vi "Main.vi"(7 "sweep rate, /min":dbl=0.2, 8 "sweep to:":dbl=-0.5, 9 "sweep":T3(radio)=enum."time_sweep") -> ()   [LabVIEW 2017] (continued)
                    n3022 = property on="2336A_addr_step" class="VISAName"() -> ("Value"=w3898:refnum<visa-resource-name>)  [unwired: 2 in, 2 out]
                    n3023 = Subtract(x=w3897, y=w3899) -> (x-y=w3900:dbl)
                    n3024 = Divide(x=w3900, y=w3896) -> (x/y=w3901:dbl)
                    n3025 = for {
                      N: w3896 -> [_]
                      tunnel: w3899 -> [w3911]
                      tunnel: w3901 -> [w3910]
                      tunnel: w3898 -> [w3907]
                      i -> [w3906]
                      n3026 = Increment(x=w3906) -> (x+1=w3905:i32)
                      n3027 = Multiply(x=w3910, y=w3905) -> (x*y=w3909:dbl)
                      n3028 = Add(x=w3909, y=w3911) -> (x+y=w3902:dbl)
                      n3029 = call "setLevel.vi"("VISA resource name 2"=w3907, "Source"=Source."Voltage", "Channel"=Channel."a", "SourceLevel"=w3902) -> ("VISA resource name"=w3903:refnum<visa-resource-name>)  [unwired: 1 in, 2 out]
                      n3030 = Wait (ms)(milliseconds to wait=u32 12) -> ()  [unwired: 1 out]
                      n3031 = property on="Current Step Value" class="DigNum (strict)"("Value"=w3902) -> ()  [unwired: 2 in, 2 out]
                      n3032 = case shown="True" "diagonal step" {
                        tunnel: w3902 -> [_ w3921]
                        tunnel: w3903 -> [_ w3914]
                        frame False {
                        }
                        frame True {
                          n3033 = Multiply(x=w3921, y="Step Slope") -> (x*y=w3919:dbl)
                          n3034 = Add(x=w3919, y="Step Offset") -> (x+y=w3915:dbl)
                          n3035 = call "setLevel.vi"("VISA resource name 2"=w3914, "Source"=Source."Voltage", "Channel"=Channel."b", "SourceLevel"=w3915) -> ()  [unwired: 1 in, 3 out]
                        }
                      }
                    }
                  }
                  frame "Radio Selection 5" {
                    # "sweep voltage on 2636a smua"
                    n3036 = property on="Step Channel" class="DigNum (strict)"() -> ("Value"=w3925:dbl)  [unwired: 2 in, 2 out]
                    n3037 = property on="Mini steps" class="DigNum (strict)"() -> ("Value"=w3922:dbl)  [unwired: 2 in, 2 out]
                    n3038 = property on="2336A_addr_step" class="VISAName"() -> ("Value"=w3924:refnum<visa-resource-name>)  [unwired: 2 in, 2 out]
                    n3039 = Subtract(x=w3923, y=w3925) -> (x-y=w3926:dbl)
                    n3040 = Divide(x=w3926, y=w3922) -> (x/y=w3927:dbl)
                    n3041 = for {
                      N: w3922 -> [_]
                      tunnel: w3925 -> [w3937]
                      tunnel: w3927 -> [w3936]
                      tunnel: w3924 -> [w3933]
                      i -> [w3932]
                      n3042 = Increment(x=w3932) -> (x+1=w3931:i32)
                      n3043 = Multiply(x=w3936, y=w3931) -> (x*y=w3935:dbl)
                      n3044 = Add(x=w3935, y=w3937) -> (x+y=w3929:dbl)
                      n3045 = call "setLevel.vi"("VISA resource name 2"=w3933, "Source"=Source."Voltage", "Channel"=Channel."b", "SourceLevel"=w3929) -> ("VISA resource name"=w3930:refnum<visa-resource-name>)  [unwired: 1 in, 2 out]
                      n3046 = Wait (ms)(milliseconds to wait=u32 12) -> ()  [unwired: 1 out]
                      n3047 = property on="diagonal step" class="Bool (strict)"() -> ("Value"=w3928:bool)  [unwired: 2 in, 2 out]
                      n3048 = property on="Current Step Value" class="DigNum (strict)"("Value"=w3929) -> ()  [unwired: 2 in, 2 out]
                      n3049 = case shown="True" w3928 {
                        tunnel: w3929 -> [_ w3947]
                        tunnel: w3930 -> [_ w3942]
                        frame False {
                        }
                        frame True {
                          n3050 = property on="Step Slope" class="DigNum (strict)"() -> ("Value"=w3941:dbl)  [unwired: 2 in, 2 out]
                          n3051 = property on="Step Offset" class="DigNum (strict)"() -> ("Value"=w3940:dbl)  [unwired: 2 in, 2 out]
                          n3052 = Multiply(x=w3947, y=w3941) -> (x*y=w3946:dbl)
                          n3053 = Add(x=w3946, y=w3940) -> (x+y=w3943:dbl)
                          n3054 = call "setLevel.vi"("VISA resource name 2"=w3942, "Source"=Source."Voltage", "Channel"=Channel."a", "SourceLevel"=w3943) -> ()  [unwired: 1 in, 3 out]
                        }
                      }
                    }
                  }
                  frame "Radio Selection 6", Default {
                    # "do not sweep, just time"
                  }
                  frame "Radio Selection 7" {
                    # "step magnetic field"
                    n3055 = stacked-sequence {
                      tunnel: w3948 -> [w3954 w3961 _]
                      frame #0 {
                        # "go to setpoint"
                        n3056 = Number To Decimal String(number="IPS120-10 addr_Step") -> (decimal integer string=w3949:string)  [unwired: 1 in]
                        n3057 = Number To Fractional String(number=w3954, width (-)=6, precision (6)=3) -> (F-format string=w3958:string)  [unwired: 1 in]
                        n3058 = Concatenate Strings("$J ", w3958) -> (w3957:string)
                        n3059 = GPIB Write(0:w3949, 1:w3957, 2:1) -> (6:w3950:errorcluster)  [unwired: 2 in, 1 out]
                        n3060 = GPIB Write(0:w3949, 1:"$A1", 2:1, 3:w3950) -> ()  [unwired: 1 in, 2 out]
                      }
                      frame #1 {
                        n3061 = while {
                          tunnel: w3961 -> [w3966]
                          stop <- w3962 stop-if-true
                          w3974 = 1
                          n3062 = local read "IPS120-10 addr_Step"() -> (w3969:u8)
                          n3063 = Number To Decimal String(number=w3969) -> (decimal integer string=w3975:string)  [unwired: 1 in]
                          n3064 = GPIB Write(0:w3975, 1:"R 7", 2:w3974) -> (6:w3970:errorcluster)  [unwired: 2 in, 1 out]
                          n3065 = GPIB Read(0:w3975, 1:200, 2:w3974, 3:w3970) -> (5:w3973:string)  [unwired: 1 in, 2 out]
                          n3066 = Fract/Exp String To Number(string=w3973, offset=w3974) -> (number=w3967:dbl)  [unwired: 2 in, 1 out]
                          n3067 = Wait (ms)(milliseconds to wait=u32 500) -> ()  [unwired: 1 out]
                          n3068 = Subtract(x=w3967, y=w3966) -> (x-y=w3965:dbl)
                          n3069 = Absolute Value(x=w3965) -> (abs(x)=w3964:dbl)
                          n3070 = Less Or Equal?(x=w3964, y=0.01) -> (x <= y?=w3962:bool)
                          "at field" <- w3962
                        }
                      }
                      frame #2 {
                        n3071 = Wait (ms)(milliseconds to wait=u32 5000) -> ()  [unwired: 1 out]
                      }
                    }
                  }
                  frame "Radio Selection 8" {
                    # "step temperature"
                    n3072 = stacked-sequence {
                      tunnel: w3977 -> [w3980 w3987]
                      frame #0 {
                        n3073 = Number To Decimal String(number="ITC503S addr_step") -> (decimal integer string=w3979:string)  [unwired: 1 in]
                        n3074 = Number To Fractional String(number=w3980, width (-)=5, precision (6)=4) -> (F-format string=w3984:string)  [unwired: 1 in]
                        n3075 = Concatenate Strings("$T ", w3984) -> (w3983:string)
                        n3076 = GPIB Write(0:w3979, 1:w3983, 2:3) -> ()  [unwired: 2 in, 2 out]
                      }
                      frame #1 {
                        n3077 = while {
                          tunnel: w3987 -> [w4003]
                          stop <- w3988 stop-if-true
                          w3994 = 1
                          n3078 = property on="ITC503S addr_step" class="DigNum (strict)"() -> ("Value"=w3990:u8)  [unwired: 2 in, 2 out]
                          n3079 = Number To Decimal String(number=w3990) -> (decimal integer string=w3997:string)  [unwired: 1 in]
                          n3080 = GPIB Write(0:w3997, 1:"$C3", 2:1) -> (6:w3998:errorcluster)  [unwired: 2 in, 1 out]
                          n3081 = GPIB Write(0:w3997, 1:"R3", 2:w3994, 3:w3998) -> (6:w4000:errorcluster)  [unwired: 1 in, 1 out]
                          n3082 = GPIB Read(0:w3997, 1:200, 2:w3994, 3:w4000) -> (5:w3999:string)  [unwired: 1 in, 2 out]
                          n3083 = Wait (ms)(milliseconds to wait=u32 500) -> ()  [unwired: 1 out]
                          n3084 = Fract/Exp String To Number(string=w3999, offset=w3994) -> (number=w3991:dbl)  [unwired: 2 in, 1 out]
                          n3085 = property on="Tolerance_Step" class="DigNum (strict)"() -> ("Value"=w3989:dbl)  [unwired: 2 in, 2 out]
                          n3086 = Subtract(x=w3991, y=w4003) -> (x-y=w4002:dbl)
                          n3087 = Absolute Value(x=w4002) -> (abs(x)=w4001:dbl)
                          n3088 = Less Or Equal?(x=w4001, y=w3989) -> (x <= y?=w3988:bool)
                          n3089 = property on="at field" class="Bool (strict)"("Value"=w3988) -> ()  [unwired: 2 in, 2 out]
                        }
                      }
                    }
                  }
                }
              }
              frame #1 {
                n3090 = property on="Current Step Value" class="DigNum (strict)"() -> ("Value"=w4008:dbl)  [unwired: 2 in, 2 out]
                n3091 = property on="Step Channel" class="DigNum (strict)"("Value"=w4008) -> ()  [unwired: 2 in, 2 out]
                n3092 = property on="Wait Between Step(s)" class="DigNum (strict)"() -> ("Value"=w4007:i32)  [unwired: 2 in, 2 out]
                n3093 = Multiply(x=w4007, y=1000) -> (x*y=w4005:i32)
                n3094 = Wait (ms)(milliseconds to wait=w4005) -> ()  [unwired: 1 out]
              }
              frame #2 {
                n3095 = Enqueue Element(queue=w4010, element="Start Sweep") -> ()  [unwired: 2 in, 3 out]
              }
            }
          }
          frame True {
            # "When step values are all finished"
            n3096 = Enqueue Element(queue=w4016, element="Idle") -> ()  [unwired: 2 in, 3 out]
            n3097 = property on="Start Mapping" class="Bool"("DisabledEnum"=T5."Enabled" ("Disabled")) -> ()  [unwired: 2 in, 2 out]
            n3098 = property on="Stop Mapping" class="Bool"("DisabledEnum"=T5."Disabled and Grayed Out" ("Disabled")) -> ()  [unwired: 2 in, 2 out]
            n3099 = property on="Sweep Direction" class="Str"("Value"="Finished!" ("Sweep Direction"), "Text.TextColor"=u32 16711680 ("Text.Text Colors:Text Color")) -> ()  [unwired: 2 in, 2 out]
          }
        }
      }
      frame "Quit" {
      }
    }
  }
  n3100 = while {
    tunnel: w3 -> [w4021]
    tunnel: w2 -> [w4019]
    tunnel: w1 -> [w4018]
    stop <- w4020 stop-if-true
    # "This loop is the producer loop."
    n3101 = event shown="[2] \"Linetrace or Mapping?\": Value Change" {
      selector: _ -> [_ _ _ _ _ _ _ _ _ _ _ _ _ _]
      dyn-events: _ -> [_ _ _ _ _ _ _ _ _ _ _ _ _ _]
      timeout: _ -> [_ _ _ _ _ _ _ _ _ _ _ _ _ _]
      tunnel: w4021 -> [_ w4023 _ w4033 _ _ w4136 w4139 w4146 w4154 w4159 w4163 _ _]
      tunnel: [_ _ _ "Quit" _ _ _ _ _ _ _ _ _ _] -> w4020
      tunnel: w4019 -> [_ _ _ _ _ _ _ _ _ _ _ _ _ _]
      tunnel: w4018 -> [_ _ _ _ _ _ _ _ _ _ _ _ _ w4203]
      event Timeout {
        n3102 = event-data() -> ()  [unwired: 1 in, 3 out]
      }
      event "Initialize": Value Change {
        n3103 = event-data() -> ()  [unwired: 1 in, 6 out]
        n3104 = Enqueue Element(queue=w4023, element="Idle") -> ()  [unwired: 2 in, 3 out]
      }
      event "Linetrace or Mapping?": Value Change {
        n3105 = event-data() -> ()  [unwired: 1 in, 1 out]
        n3106 = case shown="False" "Linetrace or Mapping?" {
          frame True {
            w4025 = T5."Enabled" ("Disabled")
            w4026 = T5."Disabled and Grayed Out" ("Disabled")
            n3107 = property on="Ramp\n Down" class="Bool"("DisabledEnum"=w4026) -> ()  [unwired: 2 in, 2 out]
            n3108 = property on="sweep" class="RadioBtnsControl (strict)"("DisabledEnum"=w4026) -> ()  [unwired: 2 in, 2 out]
            n3109 = property on="2182A 1 addr" class="DigNum (strict)"("DisabledEnum"=w4026) -> ()  [unwired: 2 in, 2 out]
            n3110 = property on="2182A 2 addr" class="DigNum (strict)"("DisabledEnum"=w4026) -> ()  [unwired: 2 in, 2 out]
            n3111 = property on="2182A 3 addr" class="DigNum (strict)"("DisabledEnum"=w4026) -> ()  [unwired: 2 in, 2 out]
            n3112 = property on="2182A 4 addr" class="DigNum (strict)"("DisabledEnum"=w4026) -> ()  [unwired: 2 in, 2 out]
            n3113 = property on="2400 1 addr" class="DigNum (strict)"("DisabledEnum"=w4026) -> ()  [unwired: 2 in, 2 out]
            n3114 = property on="IPS120-0 addr_sweep" class="DigNum (strict)"("DisabledEnum"=w4026) -> ()  [unwired: 2 in, 2 out]
            n3115 = property on="iTC_503_addr_sweep" class="DigNum (strict)"("DisabledEnum"=w4026) -> ()  [unwired: 2 in, 2 out]
            n3116 = property on="Sweep Down" class="Bool"("DisabledEnum"=w4026) -> ()  [unwired: 2 in, 2 out]
            n3117 = property on="SR830 2 addr" class="DigNum (strict)"("DisabledEnum"=w4026) -> ()  [unwired: 2 in, 2 out]
            n3118 = property on="SR830 3 addr" class="DigNum (strict)"("DisabledEnum"=w4026) -> ()  [unwired: 2 in, 2 out]
            n3119 = property on="2400 2 addr" class="DigNum (strict)"("DisabledEnum"=w4026) -> ()  [unwired: 2 in, 2 out]
            n3120 = property on="2400 3 addr" class="DigNum (strict)"("DisabledEnum"=w4026) -> ()  [unwired: 2 in, 2 out]
            n3121 = property on="2336A addr" class="VISAName"("DisabledEnum"=w4026) -> ()  [unwired: 2 in, 2 out]
            n3122 = property on="SR830 1 addr" class="DigNum (strict)"("DisabledEnum"=w4026) -> ()  [unwired: 2 in, 2 out]
            n3123 = property on="SR830 4 addr" class="DigNum (strict)"("DisabledEnum"=w4026) -> ()  [unwired: 2 in, 2 out]
            n3124 = property on="Ramp \nUp" class="Bool"("DisabledEnum"=w4026) -> ()  [unwired: 2 in, 2 out]
            n3125 = property on="Sweep Up" class="Bool"("DisabledEnum"=w4026) -> ()  [unwired: 2 in, 2 out]
            n3126 = property on="Tolerance_Sweep" class="DigNum (strict)"("DisabledEnum"=w4026) -> ()  [unwired: 2 in, 2 out]
            n3127 = property on="Continuous Sweep" class="Bool (strict)"("DisabledEnum"=w4026) -> ()  [unwired: 2 in, 2 out]
            n3128 = property on="Continuous Sweep" class="Bool (strict)"("Value"=FALSE ("Continuous Sweep")) -> ()  [unwired: 2 in, 2 out]
            n3129 = property on="MappingName" class="Str"("Visible"=TRUE) -> ()  [unwired: 2 in, 2 out]
            n3130 = property on="step" class="RadioBtnsControl (strict)"("DisabledEnum"=w4025) -> ()  [unwired: 2 in, 2 out]
            n3131 = property on="diagonal step" class="Bool (strict)"("DisabledEnum"=w4025) -> ()  [unwired: 2 in, 2 out]
            n3132 = property on="Step Offset" class="DigNum (strict)"("DisabledEnum"=w4025) -> ()  [unwired: 2 in, 2 out]
            n3133 = property on="Step Slope" class="DigNum (strict)"("DisabledEnum"=w4025) -> ()  [unwired: 2 in, 2 out]
            n3134 = property on="FieldRate(T/min)" class="DigNum (strict)"("DisabledEnum"=w4025) -> ()  [unwired: 2 in, 2 out]
            n3135 = property on="wait between sweeps(s)" class="DigNum (strict)"("DisabledEnum"=w4025) -> ()  [unwired: 2 in, 2 out]
            n3136 = property on="2336A_addr_step" class="VISAName"("DisabledEnum"=w4025) -> ()  [unwired: 2 in, 2 out]
            n3137 = property on="Start Mapping" class="Bool"("DisabledEnum"=w4025) -> ()  [unwired: 2 in, 2 out]
            n3138 = property on="2400_1_addr_step" class="DigNum (strict)"("DisabledEnum"=w4025) -> ()  [unwired: 2 in, 2 out]
            n3139 = property on="Tolerance_Step" class="DigNum (strict)"("DisabledEnum"=w4025) -> ()  [unwired: 2 in, 2 out]
            n3140 = property on="Wait Between Step(s)" class="DigNum (strict)"("DisabledEnum"=w4025) -> ()  [unwired: 2 in, 2 out]
            n3141 = property on="2400_2_addr_step" class="DigNum (strict)"("DisabledEnum"=w4025) -> ()  [unwired: 2 in, 2 out]
            n3142 = property on="IPS120-10 addr_Step" class="DigNum (strict)"("DisabledEnum"=w4025) -> ()  [unwired: 2 in, 2 out]
            n3143 = property on="ITC503S addr_step" class="DigNum (strict)"("DisabledEnum"=w4025) -> ()  [unwired: 2 in, 2 out]
          }
          frame False {
            w4029 = T5."Disabled and Grayed Out" ("Disabled")
            w4030 = T5."Enabled" ("Disabled")
            n3144 = property on="Ramp\n Down" class="Bool"("DisabledEnum"=w4030) -> ()  [unwired: 2 in, 2 out]
            n3145 = property on="sweep" class="RadioBtnsControl (strict)"("DisabledEnum"=w4030) -> ()  [unwired: 2 in, 2 out]
            n3146 = property on="2182A 1 addr" class="DigNum (strict)"("DisabledEnum"=w4030) -> ()  [unwired: 2 in, 2 out]
            n3147 = property on="2182A 2 addr" class="DigNum (strict)"("DisabledEnum"=w4030) -> ()  [unwired: 2 in, 2 out]
            n3148 = property on="2182A 3 addr" class="DigNum (strict)"("DisabledEnum"=w4030) -> ()  [unwired: 2 in, 2 out]
            n3149 = property on="2182A 4 addr" class="DigNum (strict)"("DisabledEnum"=w4030) -> ()  [unwired: 2 in, 2 out]
            n3150 = property on="2400 1 addr" class="DigNum (strict)"("DisabledEnum"=w4030) -> ()  [unwired: 2 in, 2 out]
            n3151 = property on="IPS120-0 addr_sweep" class="DigNum (strict)"("DisabledEnum"=w4030) -> ()  [unwired: 2 in, 2 out]
            n3152 = property on="iTC_503_addr_sweep" class="DigNum (strict)"("DisabledEnum"=w4030) -> ()  [unwired: 2 in, 2 out]
            n3153 = property on="Sweep Down" class="Bool"("DisabledEnum"=w4030) -> ()  [unwired: 2 in, 2 out]
            n3154 = property on="SR830 2 addr" class="DigNum (strict)"("DisabledEnum"=w4030) -> ()  [unwired: 2 in, 2 out]
            n3155 = property on="SR830 3 addr" class="DigNum (strict)"("DisabledEnum"=w4030) -> ()  [unwired: 2 in, 2 out]
            n3156 = property on="2400 2 addr" class="DigNum (strict)"("DisabledEnum"=w4030) -> ()  [unwired: 2 in, 2 out]
            n3157 = property on="2400 3 addr" class="DigNum (strict)"("DisabledEnum"=w4030) -> ()  [unwired: 2 in, 2 out]
            n3158 = property on="2336A addr" class="VISAName"("DisabledEnum"=w4030) -> ()  [unwired: 2 in, 2 out]
            n3159 = property on="SR830 1 addr" class="DigNum (strict)"("DisabledEnum"=w4030) -> ()  [unwired: 2 in, 2 out]
            n3160 = property on="SR830 4 addr" class="DigNum (strict)"("DisabledEnum"=w4030) -> ()  [unwired: 2 in, 2 out]
            n3161 = property on="Ramp \nUp" class="Bool"("DisabledEnum"=w4030) -> ()  [unwired: 2 in, 2 out]
            n3162 = property on="Sweep Up" class="Bool"("DisabledEnum"=w4030) -> ()  [unwired: 2 in, 2 out]
            n3163 = property on="Tolerance_Sweep" class="DigNum (strict)"("DisabledEnum"=w4030) -> ()  [unwired: 2 in, 2 out]
            n3164 = property on="Continuous Sweep" class="Bool (strict)"("DisabledEnum"=w4030) -> ()  [unwired: 2 in, 2 out]
            n3165 = property on="MappingName" class="Str"("Visible"=FALSE) -> ()  [unwired: 2 in, 2 out]
            n3166 = property on="step" class="RadioBtnsControl (strict)"("DisabledEnum"=w4029) -> ()  [unwired: 2 in, 2 out]
            n3167 = property on="diagonal step" class="Bool (strict)"("DisabledEnum"=w4029) -> ()  [unwired: 2 in, 2 out]
            n3168 = property on="Step Offset" class="DigNum (strict)"("DisabledEnum"=w4029) -> ()  [unwired: 2 in, 2 out]
            n3169 = property on="Step Slope" class="DigNum (strict)"("DisabledEnum"=w4029) -> ()  [unwired: 2 in, 2 out]
            n3170 = property on="wait between sweeps(s)" class="DigNum (strict)"("DisabledEnum"=w4029) -> ()  [unwired: 2 in, 2 out]
            n3171 = property on="2336A_addr_step" class="VISAName"("DisabledEnum"=w4029) -> ()  [unwired: 2 in, 2 out]
            n3172 = property on="Start Mapping" class="Bool"("DisabledEnum"=w4029) -> ()  [unwired: 2 in, 2 out]
            n3173 = property on="2400_1_addr_step" class="DigNum (strict)"("DisabledEnum"=w4029) -> ()  [unwired: 2 in, 2 out]
            n3174 = property on="Wait Between Step(s)" class="DigNum (strict)"("DisabledEnum"=w4029) -> ()  [unwired: 2 in, 2 out]
            n3175 = property on="2400_2_addr_step" class="DigNum (strict)"("DisabledEnum"=w4029) -> ()  [unwired: 2 in, 2 out]
            n3176 = property on="FieldRate(T/min)" class="DigNum (strict)"("DisabledEnum"=w4029) -> ()  [unwired: 2 in, 2 out]
            n3177 = property on="IPS120-10 addr_Step" class="DigNum (strict)"("DisabledEnum"=w4029) -> ()  [unwired: 2 in, 2 out]
            n3178 = property on="ITC503S addr_step" class="DigNum (strict)"("DisabledEnum"=w4029) -> ()  [unwired: 2 in, 2 out]
            n3179 = property on="Tolerance_Step" class="DigNum (strict)"("DisabledEnum"=w4029) -> ()  [unwired: 2 in, 2 out]
          }
        }
      }
      event "Quit": Value Change {
        n3180 = event-data() -> ()  [unwired: 1 in, 6 out]
        n3181 = Flush Queue(queue=w4033) -> (queue out=w4032:refnum<queue>)  [unwired: 1 in, 2 out]
        n3182 = Enqueue Element(queue=w4032, element="Quit") -> ()  [unwired: 2 in, 3 out]
      }
      event "Populate step table?": Value Change {
        n3183 = event-data() -> ()  [unwired: 1 in, 6 out]
        n3184 = stacked-sequence {
          frame #0 {
            n3185 = property on="Step values" class="Tbl (strict)"("Active Cell"=cluster{"Row":i32, "Column":i32} {"Row"=-2, "Column"=-2}, "Cell BG Color"=u32 16448250 ("Active Cell:Cell Background Color")) -> ()  [unwired: 2 in, 2 out]
          }
          frame #1 {
            n3186 = Subtract(x="from", y="to") -> (x-y=w4047:dbl)
            n3187 = Divide(x=w4047, y="step") -> (x/y=w4046:dbl)
            n3188 = Sign(1:w4047) -> (0:w4050:dbl)
            n3189 = Absolute Value(x=w4046) -> (abs(x)=w4045:dbl)
            n3190 = Negate(x=w4050) -> (-x=w4042:dbl)
            n3191 = Round Toward -Infinity(1:w4045) -> (0:w4044:dbl)
            n3192 = Increment(x=w4044) -> (x+1=w4043:dbl)
            n3193 = for {
              N: w4043 -> [_]
              tunnel: "from" -> [w4056]
              tunnel: w4042 -> [w4057]
              tunnel: "step" -> [w4059]
              tunnel: [w4053] -> w4048 mode=indexing
              i -> [w4051]
              n3194 = Multiply(x=w4059, y=w4051) -> (x*y=w4058:dbl)
              n3195 = Multiply(x=w4057, y=w4058) -> (x*y=w4055:dbl)
              n3196 = Add(x=w4056, y=w4055) -> (x+y=w4054:dbl)
              n3197 = Number To Fractional String(number=w4054, precision (6)=i16 6) -> (F-format string=w4053:string)  [unwired: 2 in]
            }
            n3198 = Build Array(w4048) -> (w4049:string[][])
            n3199 = Transpose 2D Array(2D array=w4049) -> (transposed array=w4041:string[][])
            n3200 = property on="Step values" class="Tbl (strict)"("Value"=w4041) -> ()  [unwired: 2 in, 2 out]
          }
          frame #2 {
            n3201 = property on="upper limit" class="DigNum (strict)"() -> ("Value"=w4089:dbl)  [unwired: 2 in, 2 out]
            n3202 = property on="lower limit" class="DigNum (strict)"() -> ("Value"=w4090:dbl)  [unwired: 2 in, 2 out]
            n3203 = Subtract(x=w4090, y=w4089) -> (x-y=w4088:dbl)
            n3204 = property on="Down Rate" class="DigNum (strict)"() -> ("Value"=w4085:dbl)  [unwired: 2 in, 2 out]
            n3205 = property on="Up Rate" class="DigNum (strict)"() -> ("Value"=w4087:dbl)  [unwired: 2 in, 2 out]
            n3206 = Absolute Value(x=w4088) -> (abs(x)=w4086:dbl)
            n3207 = property on="step" class="RadioBtnsControl (strict)"() -> ("Value"=w4061:T2)  [unwired: 2 in, 2 out]
            n3208 = Divide(x=w4086, y=w4087) -> (x/y=w4084:dbl)
            n3209 = Divide(x=w4086, y=w4085) -> (x/y=w4083:dbl)
            n3210 = case shown="\"Radio Selection 7\"" w4061 {
              tunnel: [w4091 0.0] -> w4060
              frame "Radio Selection 7" {
                n3211 = property on="step" class="DigNum (strict)"() -> ("Value"=w4095:dbl)  [unwired: 2 in, 2 out]
                n3212 = property on="FieldRate(T/min)" class="DigNum (strict)"() -> ("Value"=w4094:dbl)  [unwired: 2 in, 2 out]
                n3213 = Divide(x=w4095, y=w4094) -> (x/y=w4093:dbl)
                n3214 = Multiply(x=w4093, y=60.0) -> (x*y=w4091:dbl)
              }
              frame "Radio Selection 1".."Radio Selection 8", Default {
              }
            }
            n3215 = property on="Wait Between Step(s)" class="DigNum (strict)"() -> ("Value"=w4080:i32)  [unwired: 2 in, 2 out]
            n3216 = Add(x=w4084, y=w4083) -> (x+y=w4082:dbl)
            n3217 = Multiply(x=w4082, y=60.0) -> (x*y=w4081:dbl)
            n3218 = property on="wait between sweeps(s)" class="DigNum (strict)"() -> ("Value"=w4078:u32)  [unwired: 2 in, 2 out]
            n3219 = Add(x=w4081, y=w4080) -> (x+y=w4079:dbl)
            n3220 = property on="Step values" class="Tbl (strict)"() -> ("Value"=w4074:string[][])  [unwired: 2 in, 2 out]
            n3221 = Array Size(array=w4074) -> (size(s)=w4073:i32[])
            n3222 = Add(x=w4079, y=w4078) -> (x+y=w4063:dbl)
            n3223 = Index Array(array=w4073, index=0) -> (element=w4072:i32)
            n3224 = Add(x=w4063, y=w4060) -> (x+y=w4062:dbl)
            n3225 = Get Date/Time In Seconds() -> (seconds since 1Jan1904=w4077:timestamp)
            n3226 = Multiply(x=w4072, y=w4062) -> (x*y=w4076:dbl)
            n3227 = Add(x=w4076, y=w4077) -> (x+y=w4071:timestamp)
            n3228 = Quotient & Remainder(x=w4076, y=3600.0) -> (x-y*floor(x/y)=w4075:dbl, floor(x/y)=w4070:dbl)
            n3229 = Quotient & Remainder(x=w4075, y=60.0) -> (x-y*floor(x/y)=w4068:dbl, floor(x/y)=w4069:dbl)
            n3230 = property on="SS" class="DigNum (strict)"("Value"=w4068) -> ()  [unwired: 2 in, 2 out]
            n3231 = property on="MM:" class="DigNum (strict)"("Value"=w4069) -> ()  [unwired: 2 in, 2 out]
            n3232 = property on="HH:" class="DigNum (strict)"("Value"=w4070) -> ()  [unwired: 2 in, 2 out]
            n3233 = property on="Finish Time" class="AbsTime (strict)"("Value"=w4071) -> ()  [unwired: 2 in, 2 out]
          }
        }
      }
      event "EstimateTime": Value Change {
        n3234 = event-data() -> ()  [unwired: 1 in, 6 out]
        n3235 = property on="upper limit" class="DigNum (strict)"() -> ("Value"=w4126:dbl)  [unwired: 2 in, 2 out]
        n3236 = property on="lower limit" class="DigNum (strict)"() -> ("Value"=w4127:dbl)  [unwired: 2 in, 2 out]
        n3237 = Subtract(x=w4127, y=w4126) -> (x-y=w4125:dbl)
        n3238 = property on="Down Rate" class="DigNum (strict)"() -> ("Value"=w4122:dbl)  [unwired: 2 in, 2 out]
        n3239 = property on="Up Rate" class="DigNum (strict)"() -> ("Value"=w4124:dbl)  [unwired: 2 in, 2 out]
        n3240 = Absolute Value(x=w4125) -> (abs(x)=w4123:dbl)
        n3241 = property on="step" class="RadioBtnsControl (strict)"() -> ("Value"=w4100:T2)  [unwired: 2 in, 2 out]
        n3242 = Divide(x=w4123, y=w4124) -> (x/y=w4121:dbl)
        n3243 = Divide(x=w4123, y=w4122) -> (x/y=w4120:dbl)
        n3244 = case shown="\"Radio Selection 7\"" w4100 {
          tunnel: [w4128 0.0] -> w4098
          frame "Radio Selection 7" {
            n3245 = property on="step" class="DigNum (strict)"() -> ("Value"=w4132:dbl)  [unwired: 2 in, 2 out]
            n3246 = property on="FieldRate(T/min)" class="DigNum (strict)"() -> ("Value"=w4131:dbl)  [unwired: 2 in, 2 out]
            n3247 = Divide(x=w4132, y=w4131) -> (x/y=w4130:dbl)
            n3248 = Multiply(x=w4130, y=60.0) -> (x*y=w4128:dbl)
          }
          frame "Radio Selection 1".."Radio Selection 8", Default {
          }
        }
        n3249 = property on="Wait Between Step(s)" class="DigNum (strict)"() -> ("Value"=w4117:i32)  [unwired: 2 in, 2 out]
        n3250 = Add(x=w4121, y=w4120) -> (x+y=w4119:dbl)
        n3251 = Multiply(x=w4119, y=60.0) -> (x*y=w4118:dbl)
        n3252 = property on="wait between sweeps(s)" class="DigNum (strict)"() -> ("Value"=w4115:u32)  [unwired: 2 in, 2 out]
        n3253 = Add(x=w4118, y=w4117) -> (x+y=w4116:dbl)
        n3254 = Add(x=w4116, y=w4115) -> (x+y=w4099:dbl)
        n3255 = property on="Step values" class="Tbl (strict)"() -> ("Value"=w4108:string[][])  [unwired: 2 in, 2 out]
        n3256 = Add(x=w4099, y=w4098) -> (x+y=w4097:dbl)
        n3257 = Array Size(array=w4108) -> (size(s)=w4107:i32[])
        n3258 = Index Array(array=w4107, index=0) -> (element=w4105:i32)
        n3259 = Get Date/Time In Seconds() -> (seconds since 1Jan1904=w4114:timestamp)
        n3260 = Multiply(x=w4105, y=w4097) -> (x*y=w4113:dbl)
        n3261 = Add(x=w4113, y=w4114) -> (x+y=w4104:timestamp)
        n3262 = Quotient & Remainder(x=w4113, y=3600.0) -> (x-y*floor(x/y)=w4112:dbl, floor(x/y)=w4103:dbl)
        n3263 = Quotient & Remainder(x=w4112, y=60.0) -> (x-y*floor(x/y)=w4101:dbl, floor(x/y)=w4102:dbl)
        n3264 = property on="SS" class="DigNum (strict)"("Value"=w4101) -> ()  [unwired: 2 in, 2 out]
        n3265 = property on="MM:" class="DigNum (strict)"("Value"=w4102) -> ()  [unwired: 2 in, 2 out]
        n3266 = property on="HH:" class="DigNum (strict)"("Value"=w4103) -> ()  [unwired: 2 in, 2 out]
        n3267 = property on="Finish Time" class="AbsTime (strict)"("Value"=w4104) -> ()  [unwired: 2 in, 2 out]
      }
      event "Stop Mapping": Value Change {
        n3268 = event-data() -> ()  [unwired: 1 in, 6 out]
        n3269 = Flush Queue(queue=w4136) -> (queue out=w4137:refnum<queue>)  [unwired: 1 in, 2 out]
        n3270 = Enqueue Element(queue=w4137, element="Idle") -> ()  [unwired: 2 in, 3 out]
        n3271 = property on="Start Mapping" class="Bool"("DisabledEnum"=T5."Enabled" ("Disabled")) -> ()  [unwired: 2 in, 2 out]
        n3272 = property on="Stop Mapping" class="Bool"("DisabledEnum"=T5."Disabled and Grayed Out" ("Disabled")) -> ()  [unwired: 2 in, 2 out]
      }
      event "Sweep Down": Value Change {
        n3273 = event-data() -> ()  [unwired: 1 in, 6 out]
        n3274 = stacked-sequence {
          tunnel: w4139 -> [_ w4144]
          frame #0 {
            n3275 = property on="Down Rate" class="DigNum (strict)"() -> ("Value"=w4140:dbl)  [unwired: 2 in, 2 out]
            n3276 = property on="lower limit" class="DigNum (strict)"() -> ("Value"=w4141:dbl)  [unwired: 2 in, 2 out]
            n3277 = property on="sweep rate, /min" class="DigNum (strict)"("Value"=w4140) -> ()  [unwired: 2 in, 2 out]
            n3278 = property on="sweep to:" class="DigNum (strict)"("Value"=w4141) -> ()  [unwired: 2 in, 2 out]
            n3279 = property on="Sweep Down" class="Bool"("DisabledEnum"=T5."Disabled and Grayed Out" ("Disabled")) -> ()  [unwired: 2 in, 2 out]
          }
          frame #1 {
            n3280 = Flush Queue(queue=w4144) -> (queue out=w4143:refnum<queue>)  [unwired: 1 in, 2 out]
            n3281 = Enqueue Element(queue=w4143, element="Start Sweep") -> ()  [unwired: 2 in, 3 out]
          }
        }
      }
      event "Sweep Up": Value Change {
        n3282 = event-data() -> ()  [unwired: 1 in, 6 out]
        n3283 = stacked-sequence {
          tunnel: w4146 -> [_ w4151]
          frame #0 {
            w4147 = T5."Disabled and Grayed Out" ("Disabled")
            n3284 = property on="Up Rate" class="DigNum (strict)"() -> ("Value"=w4148:dbl)  [unwired: 2 in, 2 out]
            n3285 = property on="upper limit" class="DigNum (strict)"() -> ("Value"=w4149:dbl)  [unwired: 2 in, 2 out]
            n3286 = property on="sweep rate, /min" class="DigNum (strict)"("Value"=w4148) -> ()  [unwired: 2 in, 2 out]
            n3287 = property on="sweep to:" class="DigNum (strict)"("Value"=w4149) -> ()  [unwired: 2 in, 2 out]
            n3288 = property on="Sweep Down" class="Bool"("DisabledEnum"=w4147) -> ()  [unwired: 2 in, 2 out]
            n3289 = property on="Sweep Up" class="Bool"("DisabledEnum"=w4147) -> ()  [unwired: 2 in, 2 out]
          }
          frame #1 {
            n3290 = Flush Queue(queue=w4151) -> (queue out=w4150:refnum<queue>)  [unwired: 1 in, 2 out]
            n3291 = Enqueue Element(queue=w4150, element="Start Sweep") -> ()  [unwired: 2 in, 3 out]
          }
        }
      }
      event "Ramp\n Down": Value Change {
        n3292 = event-data() -> ()  [unwired: 1 in, 6 out]
        n3293 = Flush Queue(queue=w4154) -> (queue out=w4153:refnum<queue>)  [unwired: 1 in, 2 out]
        n3294 = property on="lower limit" class="DigNum (strict)"() -> ("Value"=w4157:dbl)  [unwired: 2 in, 2 out]
        n3295 = property on="Down Rate" class="DigNum (strict)"() -> ("Value"=w4156:dbl)  [unwired: 2 in, 2 out]
        n3296 = Enqueue Element(queue=w4153, element="Ramp To Limit") -> ()  [unwired: 2 in, 3 out]
        n3297 = property on="sweep to:" class="DigNum (strict)"("Value"=w4157) -> ()  [unwired: 2 in, 2 out]
        n3298 = property on="sweep rate, /min" class="DigNum (strict)"("Value"=w4156) -> ()  [unwired: 2 in, 2 out]
      }
      event "Ramp \nUp": Value Change {
        n3299 = event-data() -> ()  [unwired: 1 in, 6 out]
        n3300 = Flush Queue(queue=w4159) -> (queue out=w4158:refnum<queue>)  [unwired: 1 in, 2 out]
        n3301 = property on="Up Rate" class="DigNum (strict)"() -> ("Value"=w4160:dbl)  [unwired: 2 in, 2 out]
        n3302 = property on="upper limit" class="DigNum (strict)"() -> ("Value"=w4161:dbl)  [unwired: 2 in, 2 out]
        n3303 = Enqueue Element(queue=w4158, element="Ramp To Limit") -> ()  [unwired: 2 in, 3 out]
        n3304 = property on="sweep rate, /min" class="DigNum (strict)"("Value"=w4160) -> ()  [unwired: 2 in, 2 out]
        n3305 = property on="sweep to:" class="DigNum (strict)"("Value"=w4161) -> ()  [unwired: 2 in, 2 out]
      }
      event "Start Mapping": Value Change {
        n3306 = event-data() -> ()  [unwired: 1 in, 6 out]
        n3307 = stacked-sequence {
          tunnel: w4163 -> [_ _ _ w4194]
          frame #0 {
            n3308 = property on="Step values" class="Tbl (strict)"("Active Cell"=cluster{"Row":i32, "Column":i32} {"Row"=-2, "Column"=-2}, "Cell BG Color"=u32 16448250 ("Active Cell:Cell Background Color")) -> ()  [unwired: 2 in, 2 out]
          }
          frame #1 {
            n3309 = property on="lower limit" class="DigNum (strict)" props=["Value"]() -> ()  [unwired: 2 in, 3 out]
            n3310 = property on="Stop Mapping" class="Bool"("DisabledEnum"=T5."Enabled" ("Disabled")) -> ()  [unwired: 2 in, 2 out]
            n3311 = property on="upper limit" class="DigNum (strict)"() -> ("Value"=w4166:dbl)  [unwired: 2 in, 2 out]
            n3312 = property on="Down Rate" class="DigNum (strict)"() -> ("Value"=w4169:dbl)  [unwired: 2 in, 2 out]
            n3313 = property on="sweep to:" class="DigNum (strict)"("Value"=w4166) -> ()  [unwired: 2 in, 2 out]
            n3314 = property on="sweep rate, /min" class="DigNum (strict)"("Value"=w4169) -> ()  [unwired: 2 in, 2 out]
            n3315 = property on="Sweep Direction" class="Str"("Value"="Ramp Down" ("String"), "Text.TextColor"=u32 0 ("Text.Text Colors:Text Color")) -> ()  [unwired: 2 in, 2 out]
            n3316 = property on="Start Mapping" class="Bool"("DisabledEnum"=T5."Disabled and Grayed Out" ("Disabled")) -> ()  [unwired: 2 in, 2 out]
            n3317 = property on="Table Index" class="DigNum (strict)"("Value"=0.0 ("Table Index")) -> ()  [unwired: 2 in, 2 out]
          }
          frame #2 {
            # "Reserve two name strings for new mapping data file:\none for up\none for down"
            n3318 = property on="Data Folder" class="Path"() -> ("Value"=w4174:path)  [unwired: 2 in, 2 out]
            n3319 = stacked-sequence {
              tunnel: w4174 -> [w4179 w4188]
              tunnel: "MappingName" -> [w4177 w4186]
              frame #0 {
                # "Up mapping"
                n3320 = Concatenate Strings(w4177, "_up") -> (w4175:string)
                n3321 = call "AutoNamerDatExtraArtem.vi"("SweepType"=w4175, "Custom User Path"=w4179) -> ("String"=w4182:string, "Path"=w4183:path)  [unwired: 2 in]
                n3322 = Path To String(path=w4183) -> (string=w4181:string)
                n3323 = Concatenate Strings(w4181, "\\", w4182) -> (→"UpNameString":string)
              }
              frame #1 {
                # "Down mapping"
                n3324 = Concatenate Strings(w4186, "_down") -> (w4184:string)
                n3325 = call "AutoNamerDatExtraArtem.vi"("SweepType"=w4184, "Custom User Path"=w4188) -> ("String"=w4191:string, "Path"=w4192:path)  [unwired: 2 in]
                n3326 = Path To String(path=w4192) -> (string=w4190:string)
                n3327 = Concatenate Strings(w4190, "\\", w4191) -> (→"DownNameString":string)
              }
            }
          }
          frame #3 {
            n3328 = Flush Queue(queue=w4194) -> (queue out=w4193:refnum<queue>)  [unwired: 1 in, 2 out]
            n3329 = Enqueue Element(queue=w4193, element="Ramp To Limit") -> ()  [unwired: 2 in, 3 out]
          }
        }
      }
      event "Monitor": Value Change {
        n3330 = event-data() -> ()  [unwired: 1 in, 6 out]
        n3331 = case shown="False" "Monitor" {
          frame True {
            w4197 = TRUE ("Visible")
            n3332 = property on="Figure_axis" class="Arr (strict)"("Visible"=w4197) -> ()  [unwired: 2 in, 2 out]
            n3333 = property on="data" class="Arr (strict)"("Visible"=w4197) -> ()  [unwired: 2 in, 2 out]
            n3334 = property on="formula_variables" class="Arr (strict)"("Visible"=w4197) -> ()  [unwired: 2 in, 2 out]
          }
          frame False {
            w4198 = FALSE ("Visible")
            n3335 = property on="Figure_axis" class="Arr (strict)"("Visible"=w4198) -> ()  [unwired: 2 in, 2 out]
            n3336 = property on="formula_variables" class="Arr (strict)"("Visible"=w4198) -> ()  [unwired: 2 in, 2 out]
            n3337 = property on="data" class="Arr (strict)"("Visible"=w4198) -> ()  [unwired: 2 in, 2 out]
          }
        }
      }
      event "Lockin_Setup", "Cytec_Switch": Value Change {
        n3338 = event-data() -> ("CtlRef"=w4205:refnum<vi>)  [unwired: 1 in, 5 out]
        n3339 = property class="Bool"(reference=w4205) -> ("Label.Text"=w4204:string)  [unwired: 1 in, 2 out]
        n3340 = case shown="\"Cytec_Switch\", Default" w4204 {
          tunnel: w4203 -> [w4210 w4212]
          tunnel: [w4209 w4211] -> w4202
          frame "Cytec_Switch", Default {
            n3341 = Unbundle(w4210) -> ("vi reference"=w4209:refnum<vi>)  [unwired: 1 out]
          }
          frame "Lockin_Setup" {
            n3342 = Unbundle(w4212) -> ("vi reference"=w4211:refnum<vi>)  [unwired: 1 out]
          }
        }
        n3343 = invoke class="VI" method="FP.Open"(reference=w4202, "Activate"=TRUE ("Activate?")) -> (reference out=w4200:refnum<vi>)  [unwired: 3 in, 4 out]
        n3344 = property class="VI"(reference=w4200) -> (reference out=w4199:refnum<vi>, "Exec.State"=w4201:T12)  [unwired: 1 in, 1 out]
        n3345 = case shown="\"Idle\"" w4201 {
          tunnel: w4199 -> [_ w4207]
          frame "Bad", Default {
          }
          frame "Idle" {
            n3346 = invoke class="VI" method="Run VI"(reference=w4207, "Wait until done"=FALSE ("Wait Until Done")) -> ()  [unwired: 3 in, 5 out]
          }
        }
      }
    }
  }
  n3347 = Release Queue(queue=w4) -> ()  [unwired: 2 in, 3 out]
